vi "SC_schleife_init_Kelvinox.vi"   [LabVIEW 2019]
uses:
  Monitors/Utility/Monitor Communication/Kelvinox/Kelvinox_Control.ctl
  Global/Global Variables/global.vi
  Instrument_Setup.vi
  Global/Global Variables/Data_Display_global.vi
types:
  T1 = typedef "Kelvinox_Status.ctl" = cluster{"V1":bool, "V2":bool, "Dump":u16, "V4":bool, "V5":bool, "V9":bool, "P1":dbl, "P2":dbl, "P3":dbl, "P4":dbl, "P5":dbl, "Turbo":bool, "Forepump":bool, "speed":dbl, "Sorb":dbl, "1K Pot":dbl, "Still":dbl, "Cold\nPlate":dbl, "MC":dbl, "4K":dbl, "Sample":dbl, "T-Setpoint":dbl, "MC Heater":dbl, "Still Heater":dbl, "Sorb Heater":dbl, "T Control active":bool, "Sorb Res":dbl, "1K Pot Res":dbl, "Still Res":dbl, "Cold Plate Res":dbl, "MC Res":dbl, "4K Res":dbl, "Sample Res":dbl, "Ramping":bool}
  T2 = typedef "Kelvinox_Control.ctl" = cluster{"T-Setpoint-Manual":dbl, "Rate (K/min)":dbl, "Change T Control Status":bool, "Emergency Stop":bool, "Set Setpoint":bool}
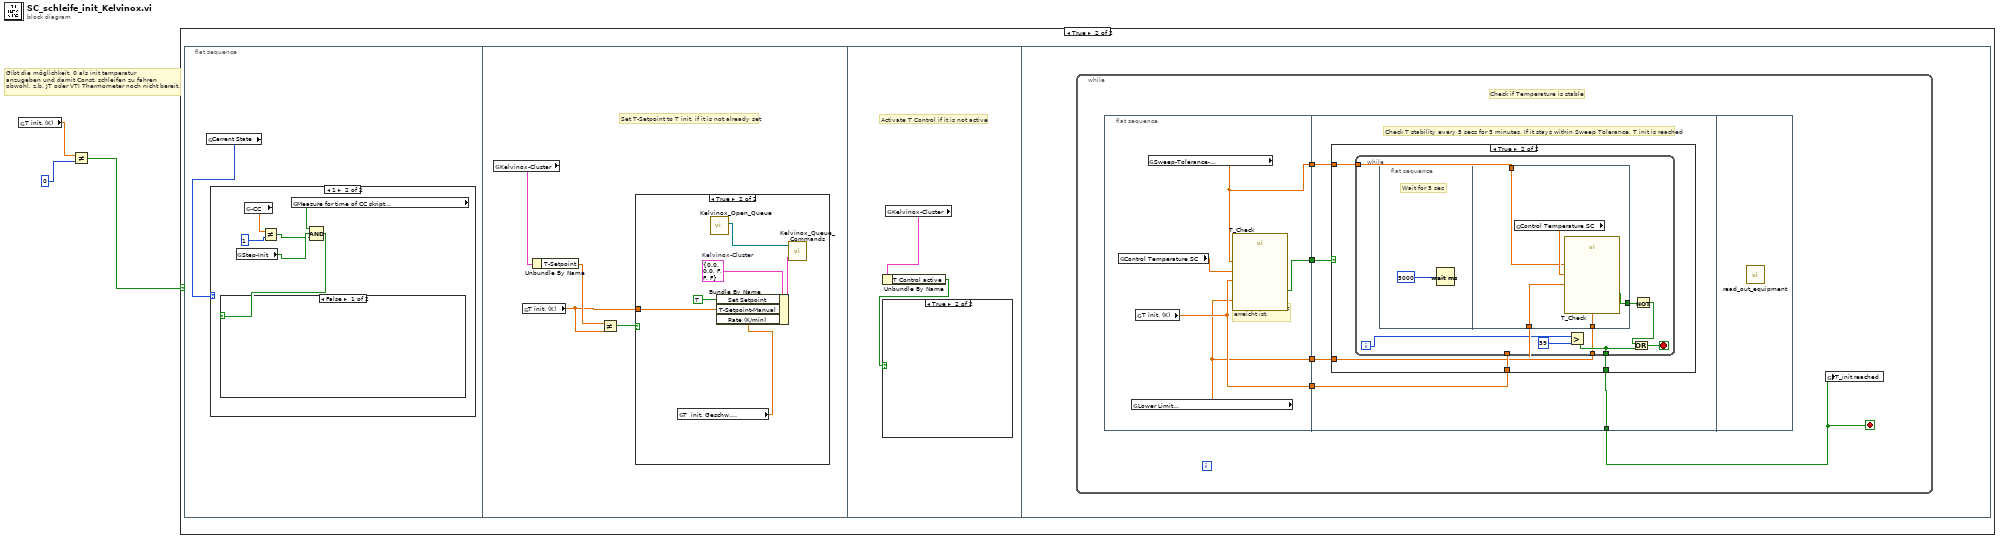
[diagram p0: block diagram]
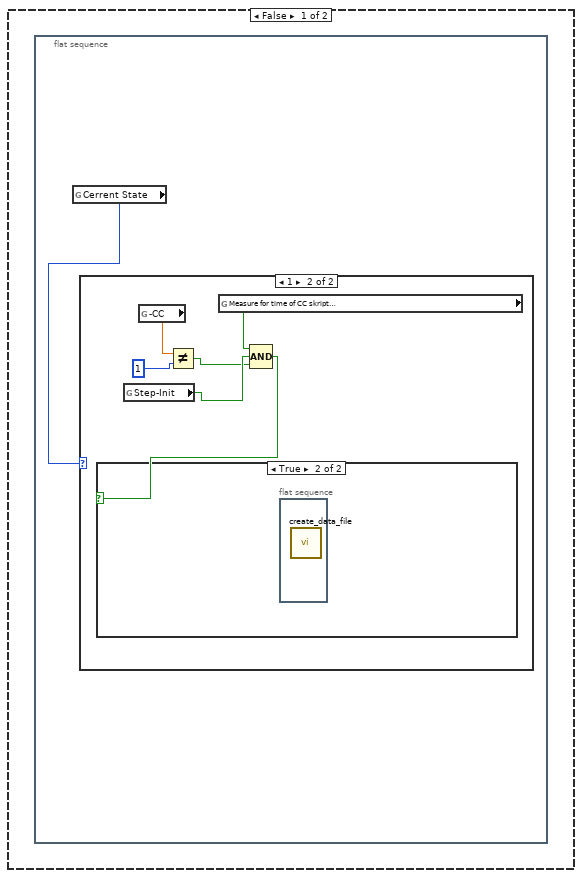
[diagram p2: hidden frame]
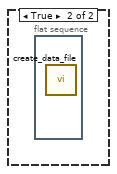
[diagram p6: hidden frame]
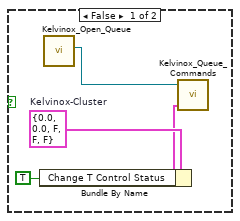
[diagram p8: hidden frame]
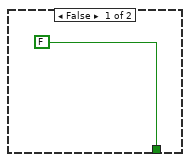
[diagram p9: hidden frame]
diagram:
  # "Gibt die möglichkeit, 0 als init temperatur \nanzugeben und damit Const. schleifen zu fahren\nobwohl, z.b. JT oder VTI Thermometer noch nicht bereit."
  n1 = global read "global.vi" "T init. (K)"() -> (w3:dbl)
  n2 = Not Equal?(x=w3, y=0) -> (x != y?=w1:bool)
  n3 = case shown="True" w1 {
    frame False {
      n4 = flat-sequence {
        frame #0 {
          n5 = global read "global.vi" "Cerrent State"() -> (w4:i32)
          n6 = case shown="1" w4 {
            frame 0, Default {
            }
            frame 1 {
              n7 = global read "global.vi" "Step-Init"() -> (w8:bool)
              n8 = global read "global.vi" "-CC"() -> (w7:dbl)
              n9 = Not Equal?(x=w7, y=1) -> (x != y?=w5:bool)
              n10 = global read "Instrument_Setup.vi" "Measure for time of CC skript\nat each field step point"() -> (w10:bool)
              n11 = Compound Arithmetic op=AND(w10, w8, w5) -> (w9:bool)
              n12 = case shown="True" w9 {
                frame False {
                }
                frame True {
                  n13 = flat-sequence {
                    frame #0 {
                      n14 = call "create_data_file.vi"() -> ()  [unwired: 3 in]
                    }
                  }
                }
              }
            }
          }
        }
      }
    }
    frame True {
      n15 = flat-sequence {
        frame #0 {
          n16 = global read "global.vi" "Cerrent State"() -> (w11:i32)
          n17 = case shown="1" w11 {
            frame 0, Default {
            }
            frame 1 {
              n18 = global read "global.vi" "Step-Init"() -> (w15:bool)
              n19 = global read "global.vi" "-CC"() -> (w14:dbl)
              n20 = Not Equal?(x=w14, y=1) -> (x != y?=w12:bool)
              n21 = global read "Instrument_Setup.vi" "Measure for time of CC skript\nat each field step point"() -> (w17:bool)
              n22 = Compound Arithmetic op=AND(w17, w15, w12) -> (w16:bool)
              n23 = case shown="False" w16 {
                frame False {
                }
                frame True {
                  n24 = flat-sequence {
                    frame #0 {
                      n25 = call "create_data_file.vi"() -> ()  [unwired: 3 in]
                    }
                  }
                }
              }
            }
          }
        }
        frame #1 {
          # "Set T-Setpoint to T init, if it is not already set"
          n26 = global read "Data_Display_global.vi" "Kelvinox-Cluster"() -> (w21:T1)
          n27 = global read "global.vi" "T init. (K)"() -> (w18:dbl)
          n28 = Unbundle By Name(w21) -> ("T-Setpoint"=w19:dbl)
          n29 = Not Equal?(x=w19, y=w18) -> (x != y?=w20:bool)
          n30 = case shown="True" w20 {
            tunnel: w18 -> [_ w23]
            frame False {
            }
            frame True {
              w26 = T2 {"T-Setpoint-Manual"=0.0, "Rate (K/min)"=0.0, "Change T Control Status"=FALSE, "Emergency Stop"=FALSE, "Set Setpoint"=FALSE}  # Kelvinox-Cluster
              n31 = global read "global.vi" "T  init. Geschw. \n(K/min)"() -> (w22:dbl)
              n32 = call "Kelvinox_Open_Queue.vi"() -> ("queue out"=w27:refnum<queue>)  [unwired: 10 in, 1 out]
              n33 = Bundle By Name(cluster=w26, "Set Setpoint"=TRUE, "T-Setpoint-Manual"=w23, "Rate (K/min)"=w22) -> (w25:T2)
              n34 = call "Kelvinox_Queue_Commands.vi"("Control"=w25, "Queue"=w27) -> ()  [unwired: 1 in, 1 out]
            }
          }
        }
        frame #2 {
          # "Activate T Control if it is not active"
          n35 = global read "Data_Display_global.vi" "Kelvinox-Cluster"() -> (w29:T1)
          n36 = Unbundle By Name(w29) -> ("T Control active"=w28:bool)
          n37 = case shown="True" w28 {
            frame False {
              w32 = T2 {"T-Setpoint-Manual"=0.0, "Rate (K/min)"=0.0, "Change T Control Status"=FALSE, "Emergency Stop"=FALSE, "Set Setpoint"=FALSE}  # Kelvinox-Cluster
              n38 = Bundle By Name(cluster=w32, "Change T Control Status"=TRUE) -> (w31:T2)
              n39 = call "Kelvinox_Open_Queue.vi"() -> ("queue out"=w33:refnum<queue>)  [unwired: 10 in, 1 out]
              n40 = call "Kelvinox_Queue_Commands.vi"("Control"=w31, "Queue"=w33) -> ()  [unwired: 1 in, 1 out]
            }
            frame True {
            }
          }
        }
        frame #3 {
          n41 = while {
            stop <- w38 stop-if-true
            # "Check if Temperature is stable"
            n42 = flat-sequence {
              tunnel: [w42] -> w37
              tunnel: [w41] -> w36
              tunnel: [w40] -> w35
              tunnel: [w39] -> w34
              tunnel: [w45] -> w38
              tunnel: w37 -> [w48]
              tunnel: w36 -> [w47]
              tunnel: w35 -> [w46]
              tunnel: w34 -> [w44]
              frame #0 {
                # "Check ob T_target\nerreicht ist."
                n43 = global read "Data_Display_global.vi" "Control Temperature SC"() -> (w43:dbl)
                n44 = global read "Instrument_Setup.vi" "Lower Limit\nSweep-Tolerance-\nTemperature (K)"() -> (w39:dbl)
                n45 = global read "global.vi" "T init. (K)"() -> (w41:dbl)
                n46 = global read "Instrument_Setup.vi" "Sweep-Tolerance-\nTemperature (%)"() -> (w40:dbl)
                n47 = call "T_Check.vi"("Lower Limit Sweep\nTolerance (K)"=w39, "T_target (K)"=w41, "Sweep\nTolerance %"=w40, "T_in"=w43) -> ("= T target"=w42:bool)
              }
              frame #1 {
                # "Check T stability every 5 secs for 5 minutes. If it stays within Sweep Tolerance, T init is reached"
                n48 = case shown="True" w48 {
                  tunnel: w47 -> [_ w53]
                  tunnel: w46 -> [_ w52]
                  tunnel: [FALSE w51] -> w45
                  tunnel: w44 -> [_ w50]
                  frame False {
                  }
                  frame True {
                    n49 = while {
                      tunnel: w53 -> [w62]
                      tunnel: w52 -> [w61]
                      tunnel: [w55] -> w51
                      tunnel: w50 -> [w54]
                      i -> [w58]
                      stop <- w59 stop-if-true
                      n50 = flat-sequence {
                        tunnel: [w67] -> w60
                        tunnel: w62 -> [w66]
                        tunnel: w61 -> [w65]
                        tunnel: w54 -> [w64]
                        frame #0 {
                          # "Wait for 5 sec"
                          n51 = Wait (ms)(milliseconds to wait=5000) -> ()  [unwired: 1 out]
                        }
                        frame #1 {
                          n52 = global read "Data_Display_global.vi" "Control Temperature SC"() -> (w68:dbl)
                          n53 = call "T_Check.vi"("Lower Limit Sweep\nTolerance (K)"=w64, "T_target (K)"=w66, "Sweep\nTolerance %"=w65, "T_in"=w68) -> ("= T target"=w67:bool)
                        }
                      }
                      n54 = Greater?(x=w58, y=59) -> (0:w55:bool)
                      n55 = Not(x=w60) -> (.not. x?=w56:bool)
                      n56 = Or(x=w56, y=w55) -> (x .or. y?=w59:bool)
                    }
                  }
                }
              }
              frame #2 {
                n57 = call "read_out_equipment.vi"() -> ()  [unwired: 1 in]
              }
            }
            n58 = global write "Data_Display_global.vi" "T_init reached"(w38) -> ()
          }
        }
      }
    }
  }
